vi "main(Test DQMH modules).vi"() -> ()   [LabVIEW 2018, in "Application.lvlib"] (continued)
              n418 = call "App enquece.vi"("command"=w959, "queue in"=w958) -> ("error out"=w960:errorcluster)  [unwired: 8 in, 1 out]
            }
            n419 = Merge Errors(w951, w949) -> (w950:errorcluster)
          }
          event "Test Channel 1": Value Change {
            n420 = event-data() -> ()  [unwired: 1 in, 1 out]
            n421 = Array Subset(array=w968, index=0, length=6) -> (w965:refnum<vi>[])
            n422 = for {
              tunnel: w965 -> [w977] mode=indexing
              n423 = property class="ColBox"(reference=w977, "Value"=u32 10000536 ("DRV 1")) -> ()  [unwired: 1 in, 2 out]
            }
            n424 = Build Array("Test Channel 1", "MEAS.AllRelaysOFF") -> (w972:string[])
            n425 = for {
              tunnel: [w981] -> w973 mode=indexing
              tunnel: w972 -> [w980] mode=indexing
              tunnel: w971 -> [w979]
              n426 = call "App enquece.vi"("command"=w980, "queue in"=w979) -> ("error out"=w981:errorcluster)  [unwired: 8 in, 1 out]
            }
            n427 = Merge Errors(w975, w973) -> (w974:errorcluster)
          }
          event "Test Channel 2": Value Change {
            n428 = event-data() -> ()  [unwired: 1 in, 1 out]
            n429 = Array Subset(array=w987, index=6, length=6) -> (w986:refnum<vi>[])
            n430 = for {
              tunnel: w986 -> [w998] mode=indexing
              n431 = property class="ColBox"(reference=w998, "Value"=u32 10000536 ("DRV 1")) -> ()  [unwired: 1 in, 2 out]
            }
            n432 = Build Array("Test Channel 2", "MEAS.AllRelaysOFF") -> (w993:string[])
            n433 = for {
              tunnel: [w1002] -> w994 mode=indexing
              tunnel: w993 -> [w1001] mode=indexing
              tunnel: w992 -> [w1000]
              n434 = call "App enquece.vi"("command"=w1001, "queue in"=w1000) -> ("error out"=w1002:errorcluster)  [unwired: 8 in, 1 out]
            }
            n435 = Merge Errors(w996, w994) -> (w995:errorcluster)
          }
          event "Test Channel 3": Value Change {
            n436 = event-data() -> ()  [unwired: 1 in, 1 out]
            n437 = Array Subset(array=w1007, index=12, length=6) -> (w1008:refnum<vi>[])
            n438 = for {
              tunnel: w1008 -> [w1019] mode=indexing
              n439 = property class="ColBox"(reference=w1019, "Value"=u32 10000536 ("DRV 1")) -> ()  [unwired: 1 in, 2 out]
            }
            n440 = Build Array("Test Channel 3", "MEAS.AllRelaysOFF") -> (w1014:string[])
            n441 = for {
              tunnel: [w1023] -> w1015 mode=indexing
              tunnel: w1014 -> [w1022] mode=indexing
              tunnel: w1013 -> [w1021]
              n442 = call "App enquece.vi"("command"=w1022, "queue in"=w1021) -> ("error out"=w1023:errorcluster)  [unwired: 8 in, 1 out]
            }
            n443 = Merge Errors(w1017, w1015) -> (w1016:errorcluster)
          }
          event "Test Channel 4": Value Change {
            n444 = event-data() -> ()  [unwired: 1 in, 1 out]
            n445 = Array Subset(array=w1028, index=18, length=6) -> (w1029:refnum<vi>[])
            n446 = for {
              tunnel: w1029 -> [w1040] mode=indexing
              n447 = property class="ColBox"(reference=w1040, "Value"=u32 10000536 ("DRV 1")) -> ()  [unwired: 1 in, 2 out]
            }
            n448 = Build Array("Test Channel 4", "MEAS.AllRelaysOFF") -> (w1035:string[])
            n449 = for {
              tunnel: [w1044] -> w1036 mode=indexing
              tunnel: w1035 -> [w1043] mode=indexing
              tunnel: w1034 -> [w1042]
              n450 = call "App enquece.vi"("command"=w1043, "queue in"=w1042) -> ("error out"=w1044:errorcluster)  [unwired: 8 in, 1 out]
            }
            n451 = Merge Errors(w1038, w1036) -> (w1037:errorcluster)
          }
          event "Test Channel 5": Value Change {
            n452 = event-data() -> ()  [unwired: 1 in, 1 out]
            n453 = Array Subset(array=w1049, index=24, length=6) -> (w1050:refnum<vi>[])
            n454 = for {
              tunnel: w1050 -> [w1061] mode=indexing
              n455 = property class="ColBox"(reference=w1061, "Value"=u32 10000536 ("DRV 1")) -> ()  [unwired: 1 in, 2 out]
            }
            n456 = Build Array("Test Channel 5", "MEAS.AllRelaysOFF") -> (w1056:string[])
            n457 = for {
              tunnel: [w1065] -> w1057 mode=indexing
              tunnel: w1056 -> [w1064] mode=indexing
              tunnel: w1055 -> [w1063]
              n458 = call "App enquece.vi"("command"=w1064, "queue in"=w1063) -> ("error out"=w1065:errorcluster)  [unwired: 8 in, 1 out]
            }
            n459 = Merge Errors(w1059, w1057) -> (w1058:errorcluster)
          }
          event "Test Channel 6": Value Change {
            n460 = event-data() -> ()  [unwired: 1 in, 1 out]
            n461 = Array Subset(array=w1070, index=30, length=6) -> (w1071:refnum<vi>[])
            n462 = for {
              tunnel: w1071 -> [w1082] mode=indexing
              n463 = property class="ColBox"(reference=w1082, "Value"=u32 10000536 ("DRV 1")) -> ()  [unwired: 1 in, 2 out]
            }
            n464 = Build Array("Test Channel 6", "MEAS.AllRelaysOFF") -> (w1077:string[])
            n465 = for {
              tunnel: [w1086] -> w1078 mode=indexing
              tunnel: w1077 -> [w1085] mode=indexing
              tunnel: w1076 -> [w1084]
              n466 = call "App enquece.vi"("command"=w1085, "queue in"=w1084) -> ("error out"=w1086:errorcluster)  [unwired: 8 in, 1 out]
            }
            n467 = Merge Errors(w1080, w1078) -> (w1079:errorcluster)
          }
          event "Test Channel 7": Value Change {
            n468 = event-data() -> ()  [unwired: 1 in, 1 out]
            n469 = Array Subset(array=w1091, index=36, length=6) -> (w1092:refnum<vi>[])
            n470 = for {
              tunnel: w1092 -> [w1103] mode=indexing
              n471 = property class="ColBox"(reference=w1103, "Value"=u32 10000536 ("DRV 1")) -> ()  [unwired: 1 in, 2 out]
            }
            n472 = Build Array("Test Channel 7", "MEAS.AllRelaysOFF") -> (w1099:string[])
            n473 = for {
              tunnel: [w1107] -> w1095 mode=indexing
              tunnel: w1099 -> [w1106] mode=indexing
              tunnel: w1098 -> [w1105]
              n474 = call "App enquece.vi"("command"=w1106, "queue in"=w1105) -> ("error out"=w1107:errorcluster)  [unwired: 8 in, 1 out]
            }
            n475 = Merge Errors(w1101, w1095) -> (w1100:errorcluster)
          }
          event "Test Channel 8": Value Change {
            n476 = event-data() -> ()  [unwired: 1 in, 1 out]
            n477 = Array Subset(array=w1112, index=42, length=6) -> (w1113:refnum<vi>[])
            n478 = for {
              tunnel: w1113 -> [w1124] mode=indexing
              n479 = property class="ColBox"(reference=w1124, "Value"=u32 10000536 ("DRV 1")) -> ()  [unwired: 1 in, 2 out]
            }
            n480 = Build Array("Test Channel 8", "MEAS.AllRelaysOFF") -> (w1119:string[])
            n481 = for {
              tunnel: [w1128] -> w1120 mode=indexing
              tunnel: w1119 -> [w1127] mode=indexing
              tunnel: w1118 -> [w1126]
              n482 = call "App enquece.vi"("command"=w1127, "queue in"=w1126) -> ("error out"=w1128:errorcluster)  [unwired: 8 in, 1 out]
            }
            n483 = Merge Errors(w1122, w1120) -> (w1121:errorcluster)
          }
          event "Test Channel 9": Value Change {
            n484 = event-data() -> ()  [unwired: 1 in, 1 out]
            n485 = Array Subset(array=w1133, index=48, length=6) -> (w1134:refnum<vi>[])
            n486 = for {
              tunnel: w1134 -> [w1145] mode=indexing
              n487 = property class="ColBox"(reference=w1145, "Value"=u32 10000536 ("DRV 1")) -> ()  [unwired: 1 in, 2 out]
            }
            n488 = Build Array("Test Channel 9", "MEAS.AllRelaysOFF") -> (w1140:string[])
            n489 = for {
              tunnel: [w1149] -> w1141 mode=indexing
              tunnel: w1140 -> [w1148] mode=indexing
              tunnel: w1139 -> [w1147]
              n490 = call "App enquece.vi"("command"=w1148, "queue in"=w1147) -> ("error out"=w1149:errorcluster)  [unwired: 8 in, 1 out]
            }
            n491 = Merge Errors(w1143, w1141) -> (w1142:errorcluster)
          }
          event "Test Channel 10": Value Change {
            n492 = event-data() -> ()  [unwired: 1 in, 1 out]
            n493 = Array Subset(array=w1154, index=54, length=6) -> (w1155:refnum<vi>[])
            n494 = for {
              tunnel: w1155 -> [w1166] mode=indexing
              n495 = property class="ColBox"(reference=w1166, "Value"=u32 10000536 ("DRV 1")) -> ()  [unwired: 1 in, 2 out]
            }
            n496 = Build Array("Test Channel 10", "MEAS.AllRelaysOFF") -> (w1161:string[])
            n497 = for {
              tunnel: [w1170] -> w1162 mode=indexing
              tunnel: w1161 -> [w1169] mode=indexing
              tunnel: w1160 -> [w1168]
              n498 = call "App enquece.vi"("command"=w1169, "queue in"=w1168) -> ("error out"=w1170:errorcluster)  [unwired: 8 in, 1 out]
            }
            n499 = Merge Errors(w1164, w1162) -> (w1163:errorcluster)
          }
          event User Event {
            n500 = event-data() -> ("Init?"=w1175:bool)  [unwired: 1 in]
            "DC Measure Module" <- w1175
            "Inst. 1" <- w1175
            n501 = disable-structure shown="LOGGING==TRUE" {
              disable-tunnel: w1178 -> [w1183 _]
              frame condition #0 (active) {
                n502 = Empty String/Path?(string/path=w1183) -> (empty?=w1189:bool)
                n503 = Select(t="Quece timeout", s=w1189, f=w1183) -> (s? t:f=w1187:string)
                n504 = Format Into String(format string=":%s", initial string=w1187, "DMM  Did  it") -> (resulting string=w1184:string)  [unwired: 1 in, 1 out]
                n505 = call "string log (SubVI).vi"("state Name"=w1184) -> ()  [unwired: 9 in, 2 out]
              }
              frame condition #1 {
              }
            }
            n506 = call "FGV Init phase.vi"("Boolean"=w1175) -> ("Init Completed?"=w1174:bool)  [unwired: 9 in, 1 out]
            n507 = case shown="True" w1174 {
              tunnel: w1173 -> [_ w1182]
              frame False {
              }
              frame True {
                n508 = call "App enquece.vi"("command"="INIT.Read DRV code", "queue in"=w1182) -> ()  [unwired: 8 in, 2 out]
              }
            }
          }
          event User Event {
            n509 = event-data() -> ("Init?"=w1193:bool)  [unwired: 1 in]
            "AC switches Module" <- w1193
            "Inst. 2" <- w1193
            n510 = disable-structure shown="LOGGING==TRUE" {
              disable-tunnel: w1198 -> [w1207 _]
              frame condition #0 (active) {
                n511 = Empty String/Path?(string/path=w1207) -> (empty?=w1213:bool)
                n512 = Select(t="Quece timeout", s=w1213, f=w1207) -> (s? t:f=w1211:string)
                n513 = Format Into String(format string=":%s", initial string=w1211, "MB01  Did  it") -> (resulting string=w1208:string)  [unwired: 1 in, 1 out]
                n514 = call "string log (SubVI).vi"("state Name"=w1208) -> ()  [unwired: 9 in, 2 out]
              }
              frame condition #1 {
              }
            }
            n515 = call "FGV Init phase.vi"("Boolean"=w1193) -> ("Init Completed?"=w1192:bool)  [unwired: 9 in, 1 out]
            n516 = case shown="True" w1192 {
              tunnel: w1191 -> [_ w1201]
              frame False {
              }
              frame True {
                n517 = call "App enquece.vi"("command"="INIT.Read DRV code", "queue in"=w1201) -> ()  [unwired: 8 in, 2 out]
              }
            }
            n518 = disable-structure shown="DEBUGGING==TRUE" {
              disable-tunnel: [w1203 w1206] -> w1197
              disable-tunnel: w1196 -> [w1203 w1205]
              frame condition #0 (active) {
              }
              frame condition #1 {
                n519 = call "Show Panel.vi"() -> ("error out"=w1204:errorcluster)  [unwired: 11 in]
                n520 = Merge Errors(w1205, w1204) -> (w1206:errorcluster)
              }
            }
          }
          event User Event {
            n521 = event-data() -> ("Init?"=w1218:bool)  [unwired: 1 in]
            "DC Switches Module" <- w1218
            "Inst. 3" <- w1218
            n522 = disable-structure shown="LOGGING==TRUE" {
              disable-tunnel: w1221 -> [w1226 _]
              frame condition #0 (active) {
                n523 = Empty String/Path?(string/path=w1226) -> (empty?=w1232:bool)
                n524 = Select(t="Quece timeout", s=w1232, f=w1226) -> (s? t:f=w1230:string)
                n525 = Format Into String(format string=":%s", initial string=w1230, "M054  Did  it") -> (resulting string=w1227:string)  [unwired: 1 in, 1 out]
                n526 = call "string log (SubVI).vi"("state Name"=w1227) -> ()  [unwired: 9 in, 2 out]
              }
              frame condition #1 {
              }
            }
            n527 = call "FGV Init phase.vi"("Boolean"=w1218) -> ("Init Completed?"=w1217:bool)  [unwired: 9 in, 1 out]
            n528 = case shown="True" w1217 {
              tunnel: w1216 -> [_ w1224]
              frame False {
              }
              frame True {
                n529 = call "App enquece.vi"("command"="INIT.Read DRV code", "queue in"=w1224) -> ()  [unwired: 8 in, 2 out]
              }
            }
          }
        }
      }
      frame "Apps.AutoMode" {
        # "Delay 1sec for Reset JIG execution Time"
        # "Check JIG trigger every 150ms"
        n530 = Wait (ms)(milliseconds to wait=u32 1000) -> ()  [unwired: 1 out]
      }
      frame "Apps.WaitingForTrigger" {
        n531 = call "App enquece.vi"("command"="MEAS.Read TRIGGER", "queue in"=w1247) -> ("error out"=w1245:errorcluster)  [unwired: 8 in, 1 out]
        n532 = Merge Errors(w1243, w1245) -> (w1244:errorcluster)
      }
      frame "Apps.UpdateStatus" {
        n533 = disable-structure shown="LOGGING==TRUE" {
          disable-tunnel: w1255 -> [w1268 _]
          frame condition #0 (active) {
            n534 = Empty String/Path?(string/path=w1268) -> (empty?=w1270:bool)
            n535 = Select(t="Quece timeout", s=w1270, f=w1268) -> (s? t:f=w1267:string)
            n536 = call "string log (SubVI).vi"("state Name"=w1267) -> ()  [unwired: 9 in, 2 out]
          }
          frame condition #1 {
          }
        }
        n537 = call "App enquece.vi"("command"="Apps.WaitForEvent", "queue in"=w1263) -> ("error out"=w1260:errorcluster)  [unwired: 8 in, 1 out]
        n538 = Merge Errors(w1256, w1260) -> (w1257:errorcluster)
      }
      frame "Apps.UI Update" {
        # "Update UI  6LED (channel)"
        n539 = disable-structure shown="LOGGING==TRUE" {
          disable-tunnel: w1274 -> [w1394 _]
          frame condition #0 (active) {
            n540 = Empty String/Path?(string/path=w1394) -> (empty?=w1396:bool)
            n541 = Select(t="Quece timeout", s=w1396, f=w1394) -> (s? t:f=w1393:string)
            n542 = call "string log (SubVI).vi"("state Name"=w1393) -> ()  [unwired: 9 in, 2 out]
          }
          frame condition #1 {
          }
        }
        n543 = Variant To Data(type="", Variant=w1272) -> (data=w1271:string)  [unwired: 1 in, 1 out]
        n544 = case shown="\"E\"" w1271 {
          tunnel: [w1295 w1303 w1321 w1339 w1357 w1375] -> w1280
          tunnel: w1278 -> [w1293 w1304 w1322 w1340 w1358 w1376]
          tunnel: w1277 -> [w1290 w1305 w1323 w1341 w1359 w1377]
          frame "", Default {
            w1287 = 6 ("length")
            n545 = call "FGV Driver Data.vi"("DUT channel (1-11)"=w1290, "FGV enum(Read)"=FGV_DRV_data."Process" ("FGV DRV data enum")) -> ("60 DRV data"=w1288:T15[])  [unwired: 6 in, 3 out]
            n546 = Decrement(x=w1290) -> (x-1=w1291:i32)
            n547 = Multiply(x=w1291, y=w1287) -> (x*y=w1289:i32)
            n548 = Array Subset(array=w1288, index=w1289, length=w1287) -> (w1286:T15[])
            n549 = Array Subset(array=w1293, index=w1289, length=w1287) -> (w1292:refnum<vi>[])
            n550 = for {
              tunnel: w1292 -> [w1298] mode=indexing
              tunnel: w1286 -> [w1297] mode=indexing
              tunnel: [w1296] -> w1295 mode=indexing
              n551 = Unbundle By Name(w1297) -> ("DRV Fail/Pass (T)"=w1301:bool)
              n552 = Select(t=u32 16711686 ("DRV 1"), s=w1301, f=u32 65309 ("DRV 1")) -> (s? t:f=w1302:u32)
              n553 = property class="ColBox"(reference=w1298, "Value"=w1302) -> (error out=w1296:errorcluster)  [unwired: 1 in, 1 out]
            }
          }
          frame "A" {
            w1306 = 1
            n554 = call "FGV Driver Data.vi"("DUT channel (1-11)"=w1305, "FGV enum(Read)"=FGV_DRV_data."Process" ("FGV DRV data enum")) -> ("60 DRV data"=w1309:T15[])  [unwired: 6 in, 3 out]
            n555 = Decrement(x=w1305) -> (x-1=w1311:i32)
            n556 = Multiply(x=w1311, y=6 ("length")) -> (x*y=w1310:i32)
            n557 = Array Subset(array=w1309, index=w1310, length=w1306) -> (w1307:T15[])
            n558 = Array Subset(array=w1304, index=w1310, length=w1306) -> (w1312:refnum<vi>[])
            n559 = for {
              tunnel: w1312 -> [w1316] mode=indexing
              tunnel: w1307 -> [w1315] mode=indexing
              tunnel: [w1314] -> w1303 mode=indexing
              n560 = Unbundle By Name(w1315) -> ("DRV Fail/Pass (T)"=w1319:bool)
              n561 = Select(t=u32 16711686 ("DRV 1"), s=w1319, f=u32 65309 ("DRV 1")) -> (s? t:f=w1320:u32)
              n562 = property class="ColBox"(reference=w1316, "Value"=w1320) -> (error out=w1314:errorcluster)  [unwired: 1 in, 1 out]
            }
          }
          frame "B" {
            w1324 = 2
            n563 = call "FGV Driver Data.vi"("DUT channel (1-11)"=w1323, "FGV enum(Read)"=FGV_DRV_data."Process" ("FGV DRV data enum")) -> ("60 DRV data"=w1327:T15[])  [unwired: 6 in, 3 out]
            n564 = Decrement(x=w1323) -> (x-1=w1329:i32)
            n565 = Multiply(x=w1329, y=6 ("length")) -> (x*y=w1328:i32)
            n566 = Array Subset(array=w1327, index=w1328, length=w1324) -> (w1325:T15[])
            n567 = Array Subset(array=w1322, index=w1328, length=w1324) -> (w1330:refnum<vi>[])
            n568 = for {
              tunnel: w1330 -> [w1334] mode=indexing
              tunnel: w1325 -> [w1333] mode=indexing
              tunnel: [w1332] -> w1321 mode=indexing
              n569 = Unbundle By Name(w1333) -> ("DRV Fail/Pass (T)"=w1337:bool)
              n570 = Select(t=u32 16711686 ("DRV 1"), s=w1337, f=u32 65309 ("DRV 1")) -> (s? t:f=w1338:u32)
              n571 = property class="ColBox"(reference=w1334, "Value"=w1338) -> (error out=w1332:errorcluster)  [unwired: 1 in, 1 out]
            }
          }
          frame "C" {
            w1342 = 3
            n572 = call "FGV Driver Data.vi"("DUT channel (1-11)"=w1341, "FGV enum(Read)"=FGV_DRV_data."Process" ("FGV DRV data enum")) -> ("60 DRV data"=w1345:T15[])  [unwired: 6 in, 3 out]
            n573 = Decrement(x=w1341) -> (x-1=w1347:i32)
            n574 = Multiply(x=w1347, y=6 ("length")) -> (x*y=w1346:i32)
            n575 = Array Subset(array=w1345, index=w1346, length=w1342) -> (w1343:T15[])
            n576 = Array Subset(array=w1340, index=w1346, length=w1342) -> (w1348:refnum<vi>[])
            n577 = for {
              tunnel: w1348 -> [w1352] mode=indexing
              tunnel: w1343 -> [w1351] mode=indexing
              tunnel: [w1350] -> w1339 mode=indexing
              n578 = Unbundle By Name(w1351) -> ("DRV Fail/Pass (T)"=w1355:bool)
              n579 = Select(t=u32 16711686 ("DRV 1"), s=w1355, f=u32 65309 ("DRV 1")) -> (s? t:f=w1356:u32)
              n580 = property class="ColBox"(reference=w1352, "Value"=w1356) -> (error out=w1350:errorcluster)  [unwired: 1 in, 1 out]
            }
          }
          frame "D" {
            w1360 = 4
            n581 = call "FGV Driver Data.vi"("DUT channel (1-11)"=w1359, "FGV enum(Read)"=FGV_DRV_data."Process" ("FGV DRV data enum")) -> ("60 DRV data"=w1363:T15[])  [unwired: 6 in, 3 out]
            n582 = Decrement(x=w1359) -> (x-1=w1365:i32)
            n583 = Multiply(x=w1365, y=6 ("length")) -> (x*y=w1364:i32)
            n584 = Array Subset(array=w1363, index=w1364, length=w1360) -> (w1361:T15[])
            n585 = Array Subset(array=w1358, index=w1364, length=w1360) -> (w1366:refnum<vi>[])
            n586 = for {
              tunnel: w1366 -> [w1370] mode=indexing
              tunnel: w1361 -> [w1369] mode=indexing
              tunnel: [w1368] -> w1357 mode=indexing
              n587 = Unbundle By Name(w1369) -> ("DRV Fail/Pass (T)"=w1373:bool)
              n588 = Select(t=u32 16711686 ("DRV 1"), s=w1373, f=u32 65309 ("DRV 1")) -> (s? t:f=w1374:u32)
              n589 = property class="ColBox"(reference=w1370, "Value"=w1374) -> (error out=w1368:errorcluster)  [unwired: 1 in, 1 out]
            }
          }
          frame "E" {
            w1378 = 5
            n590 = call "FGV Driver Data.vi"("DUT channel (1-11)"=w1377, "FGV enum(Read)"=FGV_DRV_data."Process" ("FGV DRV data enum")) -> ("60 DRV data"=w1381:T15[])  [unwired: 6 in, 3 out]
            n591 = Decrement(x=w1377) -> (x-1=w1383:i32)
            n592 = Multiply(x=w1383, y=6 ("length")) -> (x*y=w1382:i32)
            n593 = Array Subset(array=w1381, index=w1382, length=w1378) -> (w1379:T15[])
            n594 = Array Subset(array=w1376, index=w1382, length=w1378) -> (w1384:refnum<vi>[])
            n595 = for {
              tunnel: w1384 -> [w1388] mode=indexing
              tunnel: w1379 -> [w1387] mode=indexing
              tunnel: [w1386] -> w1375 mode=indexing
              n596 = Unbundle By Name(w1387) -> ("DRV Fail/Pass (T)"=w1391:bool)
              n597 = Select(t=u32 16711686 ("DRV 1"), s=w1391, f=u32 65309 ("DRV 1")) -> (s? t:f=w1392:u32)
              n598 = property class="ColBox"(reference=w1388, "Value"=w1392) -> (error out=w1386:errorcluster)  [unwired: 1 in, 1 out]
            }
          }
        }
        n599 = Merge Errors(w1281, w1280) -> (w1282:errorcluster)
      }
      frame "Apps.UI Update 1" {
        # "For Update UI 1 LED"
        n600 = disable-structure shown="LOGGING==TRUE" {
          disable-tunnel: w1411 -> [w1419 _]
          frame condition #0 (active) {
            n601 = Empty String/Path?(string/path=w1419) -> (empty?=w1421:bool)
            n602 = Select(t="Quece timeout", s=w1421, f=w1419) -> (s? t:f=w1418:string)
            n603 = call "string log (SubVI).vi"("state Name"=w1418) -> ()  [unwired: 9 in, 2 out]
          }
          frame condition #1 {
          }
        }
        n604 = call "FGV Driver Data.vi"("DUT channel (1-11)"=w1409, "FGV enum(Read)"=FGV_DRV_data."Process" ("FGV DRV data enum")) -> ("60 DRV data"=w1402:T15[])  [unwired: 6 in, 3 out]
        n605 = Decrement(x=w1397) -> (x-1=w1398:i32)
        n606 = Index Array(array=w1403, index=w1398) -> (element=w1400:refnum<vi>)
        n607 = Index Array(array=w1402, index=w1398) -> (element=w1401:T15)
        n608 = Unbundle By Name(w1401) -> ("DRV Fail/Pass (T)"=w1399:bool)
        n609 = Select(t=u32 16711686 ("DRV 1"), s=w1399, f=u32 65309 ("DRV 1")) -> (s? t:f=w1406:u32)
        n610 = property class="ColBox"(reference=w1400, "Value"=w1406) -> (error out=w1412:errorcluster)  [unwired: 1 in, 1 out]
        n611 = Merge Errors(w1413, w1412) -> (w1414:errorcluster)
      }
      frame "Apps.UI Update 2" {
        w1422 = "Test Completed!!!!"
        # "For Update PCB OK/NG (1 LED)"
        n612 = local read "Auto/Man"() -> (w1429:bool)
        n613 = disable-structure shown="LOGGING==TRUE" {
          disable-tunnel: w1441 -> [w1466 _]
          frame condition #0 (active) {
            n614 = Empty String/Path?(string/path=w1466) -> (empty?=w1468:bool)
            n615 = Select(t="Quece timeout", s=w1468, f=w1466) -> (s? t:f=w1465:string)
            n616 = call "string log (SubVI).vi"("state Name"=w1465) -> ()  [unwired: 9 in, 2 out]
          }
          frame condition #1 {
          }
        }
        n617 = case shown="True" w1429 {
          tunnel: w1434 -> [_ w1457]
          tunnel: [_ w1456] -> w1433
          frame False {
          }
          frame True {
            n618 = call "App enquece.vi"("command"="Apps.AutoMode", "queue in"=w1457) -> ("error out"=w1456:errorcluster)  [unwired: 8 in, 1 out]
          }
        }
        n619 = call "FGV DUT steps.vi"() -> ("Steps OUT"=w1427:string[])  [unwired: 11 in]
        n620 = Index Array(array=w1427, index=1) -> (element=w1428:string)
        n621 = Decimal String To Number(string=w1428) -> (number=w1425:i32)  [unwired: 2 in, 1 out]
        n622 = call "FGV Driver Data.vi"("error in (no error)"=w1433, "FGV enum(Read)"=FGV_DRV_data."Process" ("FGV DRV data enum")) -> ("error out"=w1440:errorcluster, "60 DRV data"=w1438:T15[])  [unwired: 6 in, 2 out]
        n623 = call "find Index and length.vi"("number of DRV"=w1425) -> ("length"=w1423:i32, "index"=w1424:i32)  [unwired: 8 in, 1 out]
        n624 = Array Subset(array=w1438, index=w1424, length=w1423) -> (w1431:T15[])
        n625 = for {
          tunnel: w1431 -> [w1470] mode=indexing
          tunnel: [w1469] -> w1447 mode=indexing
          n626 = Unbundle By Name(w1470) -> ("DRV Fail/Pass (T)"=w1469:bool)
        }
        n627 = control-ref of="DRV 61"() -> (w1446:refnum<vi>)
        n628 = Or Array Elements(Boolean array=w1447) -> (logical OR=w1445:bool)
        n629 = Select(t=u32 16711680 ("DRV 1"), s=w1445, f=u32 6618880 ("DRV 1")) -> (s? t:f=w1442:u32)
        n630 = property class="ColBox"(reference=w1446, error in=w1440, "Value"=w1442) -> (error out=w1439:errorcluster)  [unwired: 1 out]
        n631 = Merge Errors(w1454, w1439) -> (w1435:errorcluster)
        n632 = case shown="True" "Log report" {
          tunnel: w1431 -> [_ w1459]
          tunnel: w1430 -> [_ w1460]
          frame False {
          }
          frame True {
            # "Log trigger"
            n633 = To Variant(anything=w1459) -> (Variant=w1458:variant)
            n634 = Enqueue Element(queue=w1460, element=w1458) -> ()  [unwired: 2 in, 3 out]
          }
        }
        n635 = disable-structure shown="NO_HARDWARE==TRUE" {
          disable-tunnel: [w1461 w1464] -> w1436
          disable-tunnel: w1435 -> [w1461 w1464]
          frame condition #0 {
            n636 = Wait (ms)(milliseconds to wait=u32 2000) -> ()  [unwired: 1 out]
          }
          frame condition #1 (active) {
            n637 = Wait (ms)(milliseconds to wait=u32 20) -> ()  [unwired: 1 out]
          }
        }
        n638 = local write "Progress Status"(w1422) -> ()
      }
      frame "Apps.UI Update SC" {
        w1481 = "All Shorted Circuits"
        n639 = disable-structure shown="LOGGING==TRUE" {
          disable-tunnel: w1487 -> [w1502 _]
          frame condition #0 (active) {
            n640 = Empty String/Path?(string/path=w1502) -> (empty?=w1504:bool)
            n641 = Select(t="Quece timeout", s=w1504, f=w1502) -> (s? t:f=w1501:string)
            n642 = call "string log (SubVI).vi"("state Name"=w1501) -> ()  [unwired: 9 in, 2 out]
          }
          frame condition #1 {
          }
        }
        n643 = call "FGV DUT steps.vi"() -> ("Steps OUT"=w1474:string[])  [unwired: 11 in]
        n644 = Index Array(array=w1474, index=1) -> (element=w1476:string)
        n645 = Decimal String To Number(string=w1476) -> (number=w1475:i32)  [unwired: 2 in, 1 out]
        n646 = call "find Index and length.vi"("number of DRV"=w1475) -> ("length"=w1471:i32, "index"=w1472:i32)  [unwired: 8 in, 1 out]
        n647 = call "FGV Driver Data.vi"("FGV enum(Read)"=FGV_DRV_data."Read" ("FGV DRV data enum")) -> ("60 DRV data"=w1478:T15[])  [unwired: 7 in, 3 out]
        n648 = Array Subset(array=w1478, index=w1472, length=w1471) -> (w1477:T15[])
        n649 = Array Subset(array=w1480, index=w1472, length=w1471) -> (w1479:refnum<vi>[])
        n650 = for {
          tunnel: w1477 -> [w1511] mode=indexing
          tunnel: w1479 -> [w1506] mode=indexing
          tunnel: [w1505] -> w1485 mode=indexing
          n651 = Unbundle By Name(w1511) -> ("Shorted Circuit"=w1507:bool)
          n652 = Select(t=u32 16711680 ("DRV 1"), s=w1507, f=u32 6618880 ("DRV 1")) -> (s? t:f=w1510:u32)
          n653 = property class="ColBox"(reference=w1506, "Value"=w1510) -> (error out=w1505:errorcluster)  [unwired: 1 in, 1 out]
        }
        n654 = Merge Errors(w1485) -> (w1484:errorcluster)
        n655 = flat-sequence {
          tunnel: w1484 -> [w1497]
          tunnel: [w1497] -> w1483
          tunnel: w1483 -> [w1499]
          tunnel: [w1500] -> w1482
          tunnel: w1480 -> [w1498]
          frame #0 {
            n656 = Wait (ms)(milliseconds to wait=u32 500) -> ()  [unwired: 1 out]
          }
          frame #1 {
            n657 = call "reset DRV UI (SubVI).vi"("error in (no error)"=w1499, "Ref  in"=w1498) -> ("error out"=w1500:errorcluster)  [unwired: 8 in, 1 out]
          }
        }
        n658 = Merge Errors(w1495, w1482) -> (w1486:errorcluster)
        n659 = local write "Progress Status"(w1481) -> ()
      }
      frame "Timer Start" {
        n660 = flat-sequence {
          tunnel: [""] -> w1512
          frame #0 {
            n661 = call "FGV milisec (subVI).vi"() -> ()  [unwired: 11 in, 1 out]
          }
        }
        n662 = local write "elapsed Time"(w1512) -> ()
      }
      frame "Timer Stop" {
        n663 = flat-sequence {
          tunnel: [w1537] -> w1527
          tunnel: w1528 -> [w1537]
          tunnel: [w1536] -> w1526
          frame #0 {
            n664 = call "FGV milisec (subVI).vi"() -> ("Elased Time (ms)"=w1536:u32)  [unwired: 11 in]
          }
        }
        n665 = Format Into String(initial string="t = ", w1526) -> (resulting string=w1524:string)  [unwired: 2 in, 1 out]
        n666 = Concatenate Strings(w1524, "  [ms] " ("initial string")) -> (→"elapsed Time":string)
      }
      frame "WaitFor" {
        n667 = flat-sequence {
          tunnel: [w1547] -> w1538
          tunnel: w1539 -> [w1547]
          frame #0 {
            n668 = Wait (ms)(milliseconds to wait="wait for (ms)") -> ()  [unwired: 1 out]
          }
        }
      }
      frame "WaitForA" {
        n669 = flat-sequence {
          tunnel: [w1563] -> w1549
          tunnel: w1550 -> [w1563]
          frame #0 {
            n670 = local read "wait for (ms)"() -> (w1561:u32)
            n671 = Multiply(x=u32 230, y=u32 1) -> (x*y=w1562:u32)
            n672 = Subtract(x=w1561, y=w1562) -> (x-y=w1560:u32)
            n673 = Wait (ms)(milliseconds to wait=w1560) -> ()  [unwired: 1 out]
          }
        }
      }
      frame "WaitForB" {
        n674 = flat-sequence {
          tunnel: [w1578] -> w1564
          tunnel: w1565 -> [w1578]
          frame #0 {
            n675 = local read "wait for (ms)"() -> (w1576:u32)
            n676 = Multiply(x=u32 230, y=u32 2) -> (x*y=w1577:u32)
            n677 = Subtract(x=w1576, y=w1577) -> (x-y=w1575:u32)
            n678 = Wait (ms)(milliseconds to wait=w1575) -> ()  [unwired: 1 out]
          }
        }
      }
      frame "WaitForC" {
        n679 = flat-sequence {
          tunnel: [w1593] -> w1579
          tunnel: w1580 -> [w1593]
          frame #0 {
            n680 = local read "wait for (ms)"() -> (w1591:u32)
            n681 = Multiply(x=u32 230, y=u32 3) -> (x*y=w1592:u32)
            n682 = Subtract(x=w1591, y=w1592) -> (x-y=w1590:u32)
            n683 = Wait (ms)(milliseconds to wait=w1590) -> ()  [unwired: 1 out]
          }
        }
      }
      frame "WaitForD" {
        n684 = flat-sequence {
          tunnel: [w1608] -> w1594
          tunnel: w1595 -> [w1608]
          frame #0 {
            n685 = local read "wait for (ms)"() -> (w1606:u32)
            n686 = Multiply(x=u32 230, y=u32 4) -> (x*y=w1607:u32)
            n687 = Subtract(x=w1606, y=w1607) -> (x-y=w1605:u32)
            n688 = Wait (ms)(milliseconds to wait=w1605) -> ()  [unwired: 1 out]
          }
        }
      }
      frame "WaitForE" {
        n689 = flat-sequence {
          tunnel: [w1623] -> w1609
          tunnel: w1610 -> [w1623]
          frame #0 {
            n690 = local read "wait for (ms)"() -> (w1621:u32)
            n691 = Multiply(x=u32 230, y=u32 5) -> (x*y=w1622:u32)
            n692 = Subtract(x=w1621, y=w1622) -> (x-y=w1620:u32)
            n693 = Wait (ms)(milliseconds to wait=w1620) -> ()  [unwired: 1 out]
          }
        }
      }
      frame "Apps.Exit" {
        w1628 = TRUE
        n694 = disable-structure shown="LOGGING==TRUE" {
          disable-tunnel: w1625 -> [w1643 _]
          frame condition #0 (active) {
            n695 = Empty String/Path?(string/path=w1643) -> (empty?=w1645:bool)
            n696 = Select(t="Quece timeout", s=w1645, f=w1643) -> (s? t:f=w1642:string)
            n697 = call "string log (SubVI).vi"("state Name"=w1642) -> ()  [unwired: 9 in, 2 out]
          }
          frame condition #1 {
          }
        }
        n698 = call "Application Name--constant.vi"() -> ("Application Name"=w1629:string)  [unwired: 11 in]
        n699 = call "Stop Module.vi"("Wait for Module to Stop? (F)"=w1628, "Origin"=w1629) -> ("error out"=w1637:errorcluster)  [unwired: 9 in]
        n700 = call "Stop Module.vi"("Wait for Module to Stop? (F)"=w1628, "Origin"=w1629) -> ("error out"=w1636:errorcluster)  [unwired: 9 in]
        n701 = call "Stop Module.vi"("Wait for Module to Stop? (F)"=w1628, "Origin"=w1629) -> ("error out"=w1635:errorcluster)  [unwired: 9 in]
        n702 = call "Stop Module.vi"("Wait for Module to stop? (F)"=w1628, "Origin"=w1629, "Module ID"=-1) -> ("error out"=w1631:errorcluster)  [unwired: 8 in]
        n703 = Merge Errors(w1633, w1637, w1636, w1635, w1631) -> (w1634:errorcluster)
      }
      frame "Apps.Error Handler" {
        w1654 = TRUE  # Priority Enquece
        n704 = disable-structure shown="LOGGING==TRUE" {
          disable-tunnel: w1647 -> [w1663 _]
          frame condition #0 (active) {
            n705 = Empty String/Path?(string/path=w1663) -> (empty?=w1665:bool)
            n706 = Select(t="Quece timeout", s=w1665, f=w1663) -> (s? t:f=w1662:string)
            n707 = call "string log (SubVI).vi"("state Name"=w1662) -> ()  [unwired: 9 in, 2 out]
          }
          frame condition #1 {
          }
        }
        n708 = call <vilib>:"Simple Error Handler.vi"("error in (no error)"=w1661) -> ("error out"=w1656:errorcluster)  [unwired: 4 in, 4 out]
        n709 = flat-sequence {
          tunnel: w1656 -> [_]
          tunnel: [w1666] -> w1648
          frame #0 {
            n710 = xnode "Error Ring"() -> ("error out"=w1666:errorcluster)
          }
        }
        n711 = call "App enquece.vi"("Priority Enquece"=w1654, "command"="Apps.Exit", "queue in"=w1655) -> ("error out"=w1653:errorcluster)  [unwired: 7 in, 1 out]
        n712 = Merge Errors(w1648, w1653) -> (w1649:errorcluster)
      }
      frame "INIT.Init FGV" {
        n713 = call "FGV_HoldingRegs.vi"("FGV_enum"=FGV_enum."Init FGV") -> ("error out"=w1673:errorcluster)  [unwired: 8 in, 2 out]
        n714 = call "string log (SubVI).vi"("error in (no error)"=w1673, "Enum(log)"=enum16{"Init", "Log", "Read", "Clear"}."Init") -> ("error out"=w1674:errorcluster)  [unwired: 8 in, 1 out]
        n715 = call "FGV Driver Data.vi"("error in (no error)"=w1674, "FGV enum(Read)"=FGV_DRV_data."Init" ("FGV DRV data enum")) -> ("error out"=w1671:errorcluster)  [unwired: 6 in, 3 out]
        n716 = call "FGV Init phase.vi"("error in (no error)"=w1671, "FGV Enum"=enum16{"Init", "Check"}."Init") -> ("error out"=w1669:errorcluster)  [unwired: 8 in, 1 out]
        n717 = flat-sequence {
          tunnel: [w1686] -> w1670
          tunnel: w1669 -> [w1686]
          frame #0 {
            n718 = Initialize Array(FALSE, 6 ("dimension size"), 10 ("dimension size")) -> (w1690:bool[][])
            n719 = local write "Auto/Man"(FALSE) -> ()
            n720 = local write "EMIC connected"(bool[] [FALSE, FALSE, FALSE, FALSE, FALSE, FALSE] ("Array")) -> ()
            n721 = local write "Short DRV"(w1690) -> ()
          }
        }
        n722 = Merge Errors(w1685, w1670) -> (w1675:errorcluster)
      }
      frame "INIT.Read HW config" {
        n723 = disable-structure shown="LOGGING==TRUE" {
          disable-tunnel: w1705 -> [w1731 _]
          frame condition #0 (active) {
            n724 = Empty String/Path?(string/path=w1731) -> (empty?=w1733:bool)
            n725 = Select(t="Quece timeout", s=w1733, f=w1731) -> (s? t:f=w1730:string)
            n726 = call "string log (SubVI).vi"("state Name"=w1730) -> ()  [unwired: 9 in, 2 out]
          }
          frame condition #1 {
          }
        }
        n727 = call <vilib>:"Application Directory.vi"() -> ("Application Directory"=w1700:path)
        n728 = Build Path(base path=w1700, name or relative path="config") -> (appended path=w1699:path)
        n729 = call "HW Config.vi"("start path"=w1699) -> ("error out"=w1706:errorcluster, "HW config 2"=w1713:T7)  [unwired: 9 in]
        n730 = Bundle By Name(cluster=w1714, "HW config 2"=w1713) -> (w1712:cluster{"HW config 2":T7})
        n731 = invoke class="VI" method="FP.Open"(error in=w1706, "State"=T17."Minimized") -> (error out=w1695:errorcluster)  [unwired: 3 in, 4 out]
        n732 = call "Login.vi"("error in (no error)"=w1695) -> ("error out"=w1697:errorcluster, "Login Successed"=w1698:bool, "UserName"=w1694:string)  [unwired: 8 in]
        n733 = call "FGV _Operator Name.vi"("Enum"=enum16{"Write", "Read"}."Write", "Operator Name in"=w1694) -> ()  [unwired: 9 in, 1 out]
        n734 = case shown="True" w1698 {
          tunnel: w1702 -> [w1724 _]
          tunnel: w1697 -> [w1721 w1726]
          tunnel: [w1720 w1727] -> w1707
          frame False {
            n735 = call "string log (SubVI).vi"("Enum(log)"=enum16{"Init", "Log", "Read", "Clear"}."Init") -> ("error out"=w1719:errorcluster)  [unwired: 9 in, 1 out]
            n736 = call "App enquece.vi"("Priority Enquece"=TRUE, "error in (no error)"=w1721, "command"="Apps.Exit", "queue in"=w1724) -> ("error out"=w1720:errorcluster)  [unwired: 6 in, 1 out]
            n737 = call "inst.InitialiseFGV.vi"("error in (no error)"=w1719) -> ()  [unwired: 10 in, 1 out]
          }
          frame True {
            n738 = invoke class="VI" method="FP.Open"(error in=w1726, "State"=T17."Standard") -> (error out=w1727:errorcluster)  [unwired: 3 in, 4 out]
          }
        }
        n739 = Merge Errors(w1717, w1707) -> (w1708:errorcluster)
        n740 = disable-structure shown="RUN_TIME_ENGINE==True" {
          disable-tunnel: ["Under Development" ("version") "v5.0 Released"] -> w1704
          frame condition #0 (active) {
          }
          frame condition #1 {
          }
        }
        "version" <- w1704
      }
      frame "INIT.Read DRV code" {
        n741 = disable-structure shown="LOGGING==TRUE" {
          disable-tunnel: w1762 -> [w1795 _]
          frame condition #0 (active) {
            n742 = Empty String/Path?(string/path=w1795) -> (empty?=w1797:bool)
            n743 = Select(t="Quece timeout", s=w1797, f=w1795) -> (s? t:f=w1794:string)
            n744 = call "string log (SubVI).vi"("state Name"=w1794) -> ()  [unwired: 9 in, 2 out]
          }
          frame condition #1 {
          }
        }
        n745 = invoke class="VI" method="FP.Open"("State"=T17."Minimized") -> (error out=w1756:errorcluster)  [unwired: 4 in, 4 out]
        n746 = call "ReadDriverParameters.vi"("error in (no error)"=w1756) -> ("error out"=w1754:errorcluster, "DRV stand"=w1745:T16)  [unwired: 9 in]
        n747 = invoke class="VI" method="FP.Open"(error in=w1754, "State"=T17."Standard") -> (error out=w1758:errorcluster)  [unwired: 3 in, 4 out]
        n748 = Merge Errors(w1763, w1758) -> (w1764:errorcluster)
        n749 = call "FGV DRV stand.vi"("Enum(read)"=enum16{"Write", "Read"}."Write" ("Enum"), "DRV stand  in"=w1745) -> ("Sub-Test.DCV"=w1734:bool, "DRV stand out"=w1744:T16)  [unwired: 8 in]
        n750 = Unbundle By Name(w1744) -> ("SAP ID"=w1751:string, "Name"=w1752:string)
        "DUT Name" <- w1752
        n751 = call "FGV SapID & Name.vi"("Enum"=enum16{"Read", "Write"}."Write", "Name"=w1752, "SAP ID"=w1751) -> ("SAP ID out"=w1748:string)  [unwired: 7 in, 1 out]
        n752 = case shown="True" w1734 {
          tunnel: w1761 -> [_ w1787]
          tunnel: [_ w1774] -> w1753
          tunnel: w1744 -> [_ w1773]
          tunnel: ["HV-60D ready!!!!!!!!!!!!!!!!" w1772] -> w1747
          tunnel: w1746 -> [_ w1772]
          frame False {
          }
          frame True {
            w1786 = u8 2 items=["SLOW", "MID", "FAST"] ("Detector Rate")
            # "Convert from [mA] to [A]"
            n753 = Unbundle By Name(w1773) -> ("DC characteristics.Voltage.Max"=w1778:dbl, "DC characteristics.Current.Max"=w1793:dbl)
            n754 = Divide(x=w1793, y=1000.0) -> (x/y=w1775:dbl)
            n755 = Bundle By Name(cluster=T19 {"DMM config cluster"={"DCV range"=0.0, "DCI range"=0.0, "Detector Rate"=0}, "mux2-1(DMM I) encode"=enum."DMM I (0.5)"} ("DMM all config"), "DMM config cluster.DCV range"=w1778, "DMM config cluster.DCI range"=w1775, "DMM config cluster.Detector Rate"=w1786) -> (w1790:T19)
            n756 = Greater?(x=w1775, y=0.5) -> (0:w1776:bool)
            n757 = To Variant(anything=w1790) -> (Variant=w1789:variant)
            n758 = Select(t=enum16{"DMM I (0.5)", "DMM I (12)"}."DMM I (12)" ("mux2-1(DMM I) encode 2"), s=w1776, f=enum16{"DMM I (0.5)", "DMM I (12)"}."DMM I (0.5)" ("mux2-1(DMM I) encode 2")) -> (s? t:f=w1782:enum16{"DMM I (0.5)", "DMM I (12)"})
            n759 = call "App enquece.vi"("command data"=w1789, "command"="MEAS.Set DMM config", "queue in"=w1787) -> ("error out"=w1779:errorcluster, "Queue out"=w1783:refnum<queue>)  [unwired: 7 in]
            n760 = To Variant(anything=w1782) -> (Variant=w1784:variant)
            n761 = call "App enquece.vi"("error in (no error)"=w1779, "command data"=w1784, "command"="MEAS.Sel Input Current", "queue in"=w1783) -> ("error out"=w1774:errorcluster)  [unwired: 6 in, 1 out]
          }
        }
        n762 = call "FGV DUT steps.vi"("Enum(read)"=enum16{"write", "read"}."write" ("Enum"), "SapID"=w1748) -> ("Steps OUT"=w1740:string[])  [unwired: 9 in]
        n763 = Index Array(array=w1740, index #1=0 ("index")) -> (element #1=→"SAP ID":string, element #2=→"#DRV":string, element #3=w1735:string)  [unwired: 2 in]
        n764 = Decimal String To Number(string=w1735) -> (number=w1742:i32)  [unwired: 2 in, 1 out]
        n765 = To Unsigned Long Integer(number=w1742) -> (unsigned 32bit integer=w1741:u32)
        n766 = local write "wait for (ms)"(w1741) -> ()
        n767 = Array Subset(array=w1740, index=3) -> (→"List of Actions":string[])  [unwired: 1 in]
        n768 = Merge Errors(w1764, w1753) -> (w1760:errorcluster)
      }
      frame "INIT.Call DMM module" {
        n769 = disable-structure shown="LOGGING==TRUE" {
          disable-tunnel: w1799 -> [w1817 _]
          frame condition #0 (active) {
            n770 = Empty String/Path?(string/path=w1817) -> (empty?=w1819:bool)
            n771 = Select(t="Quece timeout", s=w1819, f=w1817) -> (s? t:f=w1816:string)
            n772 = call "string log (SubVI).vi"("state Name"=w1816) -> ()  [unwired: 9 in, 2 out]
          }
          frame condition #1 {
          }
        }
        n773 = Unbundle By Name(w1810) -> ("HW config 2.DMM"=w1809:string)
        n774 = Type Cast(type=refnum<visa-resource-name> refnum ("VISA resource name 2"), x=w1809) -> (*(type *) &x=w1807:refnum<visa-resource-name>)
        n775 = call "Start Module.vi"("VISA resource name 2"=w1807) -> ("error out"=w1812:errorcluster, "Wait for Event Sync?"=w1806:bool, "DMM Module Broadcast Events"=w1805:T13)  [unwired: 7 in, 1 out]
        n776 = register-events(reference=w1813, w1805) -> (reference out=w1814:refnum<event-registration>)  [unwired: 5 in, 1 out]
        n777 = call "Synchronize Module Events.vi"("error in"=w1812, "Wait for Event Sync?"=w1806) -> ("error out"=w1811:errorcluster)  [unwired: 9 in]
        n778 = Merge Errors(w1800, w1811) -> (w1801:errorcluster)
      }
      frame "INIT.Call MUX module" {
        n779 = disable-structure shown="LOGGING==TRUE" {
          disable-tunnel: w1821 -> [w1839 _]
          frame condition #0 (active) {
            n780 = Empty String/Path?(string/path=w1839) -> (empty?=w1841:bool)
            n781 = Select(t="Quece timeout", s=w1841, f=w1839) -> (s? t:f=w1838:string)
            n782 = call "string log (SubVI).vi"("state Name"=w1838) -> ()  [unwired: 9 in, 2 out]
          }
          frame condition #1 {
          }
        }
        n783 = Unbundle By Name(w1833) -> ("HW config 2.mux"=w1832:string)
        n784 = Type Cast(type=refnum<visa-resource-name> refnum ("VISA resource name"), x=w1832) -> (*(type *) &x=w1831:refnum<visa-resource-name>)
        n785 = call "Start Module.vi"("VISA resource name"=w1831) -> ("error out"=w1834:errorcluster, "Wait for Event Sync?"=w1828:bool, "Switches Module Broadcast Events"=w1829:T11)  [unwired: 7 in, 1 out]
        n786 = register-events(reference=w1835, w1829) -> (reference out=w1836:refnum<event-registration>)  [unwired: 5 in, 1 out]
        n787 = call "Synchronize Module Events.vi"("error in"=w1834, "Wait for Event Sync?"=w1828) -> ("error out"=w1827:errorcluster)  [unwired: 9 in]
        n788 = Merge Errors(w1822, w1827) -> (w1823:errorcluster)
      }
      frame "INIT.Call DEMUX module" {
        n789 = disable-structure shown="LOGGING==TRUE" {
          disable-tunnel: w1844 -> [w1861 _]
          frame condition #0 (active) {
            n790 = Empty String/Path?(string/path=w1861) -> (empty?=w1863:bool)
            n791 = Select(t="Quece timeout", s=w1863, f=w1861) -> (s? t:f=w1860:string)
            n792 = call "string log (SubVI).vi"("state Name"=w1860) -> ()  [unwired: 9 in, 2 out]
          }
          frame condition #1 {
          }
        }
        n793 = Unbundle By Name(w1855) -> ("HW config 2.demux"=w1854:string)
        n794 = Type Cast(type=refnum<visa-resource-name> refnum ("COMport name"), x=w1854) -> (*(type *) &x=w1853:refnum<visa-resource-name>)
        n795 = call "Start Module.vi"("COMport name"=w1853) -> ("error out"=w1856:errorcluster, "Wait for Event Sync?"=w1842:bool, "MB 01 switches Module Broadcast Events"=w1851:T12)  [unwired: 7 in, 1 out]
        n796 = register-events(reference=w1857, w1851) -> (reference out=w1858:refnum<event-registration>)  [unwired: 5 in, 1 out]
        n797 = call "Synchronize Module Events.vi"("error in"=w1856, "Wait for Event Sync?"=w1842) -> ("error out"=w1850:errorcluster)  [unwired: 9 in]
        n798 = Merge Errors(w1845, w1850) -> (w1846:errorcluster)
      }
      frame "INIT.Call EMIC modules" {
        n799 = disable-structure shown="LOGGING==TRUE" {
          disable-tunnel: w1867 -> [w1884 _]
          frame condition #0 (active) {
            n800 = Empty String/Path?(string/path=w1884) -> (empty?=w1886:bool)
            n801 = Select(t="Quece timeout", s=w1886, f=w1884) -> (s? t:f=w1883:string)
            n802 = call "string log (SubVI).vi"("state Name"=w1883) -> ()  [unwired: 9 in, 2 out]
          }
          frame condition #1 {
          }
        }
        n803 = Unbundle By Name(w1874) -> ("HW config 2.eMIC1"=w1881:string, "HW config 2.eMIC2"=w1880:string, "HW config 2.eMIC3"=w1879:string, "HW config 2.eMIC4"=w1878:string, "HW config 2.eMIC5"=w1877:string, "HW config 2.eMIC6"=w1876:string)
        n804 = Build Array(w1881, w1880, w1879, w1878, w1877, w1876) -> (w1865:string[])
        n805 = for {
          shift-right: [w1896] -> w1873
          shift-left: w1875 -> [w1894]
          tunnel: w1865 -> [w1895] mode=indexing
          tunnel: [w1888] -> w1871 mode=indexing
          n806 = Type Cast(type=refnum<visa-resource-name> refnum ("VISA resource name"), x=w1895) -> (*(type *) &x=w1892:refnum<visa-resource-name>)
          n807 = call "Start Module.vi"("VISA resource name"=w1892) -> ("error out"=w1889:errorcluster, "Wait for Event Sync?"=w1887:bool, "CE14_v2 Broadcast Events"=w1891:T10, "Module ID"=w1890:i32)  [unwired: 7 in]
          n808 = register-events(reference=w1894, w1891) -> (reference out=w1896:refnum<event-registration>)  [unwired: 5 in, 1 out]
          n809 = call "Synchronize Module Events.vi"("error in"=w1889, "Wait for Event Sync?"=w1887, "Module ID in"=w1890) -> ("error out"=w1888:errorcluster)  [unwired: 7 in, 1 out]
        }
        n810 = Merge Errors(w1868, w1871) -> (w1866:errorcluster)
      }
      frame "INIT.Open COM DMM" {
        n811 = disable-structure shown="LOGGING==TRUE" {
          disable-tunnel: w1900 -> [w1912 _]
          frame condition #0 (active) {
            n812 = Empty String/Path?(string/path=w1912) -> (empty?=w1914:bool)
            n813 = Select(t="Quece timeout", s=w1914, f=w1912) -> (s? t:f=w1911:string)
            n814 = call "string log (SubVI).vi"("state Name"=w1911) -> ()  [unwired: 9 in, 2 out]
          }
          frame condition #1 {
          }
        }
        n815 = call "DMM connect and reset.vi"() -> ("error out"=w1904:errorcluster)  [unwired: 11 in]
        n816 = Merge Errors(w1901, w1904) -> (w1898:errorcluster)
        n817 = flat-sequence {
          tunnel: [w1910] -> w1899
          tunnel: w1898 -> [w1910]
          frame #0 {
            n818 = Wait (ms)(milliseconds to wait=u32 70) -> ()  [unwired: 1 out]
          }
        }
      }
      frame "INIT.Open COM MUX" {
        n819 = disable-structure shown="LOGGING==TRUE" {
          disable-tunnel: w1918 -> [w1930 _]
          frame condition #0 (active) {
            n820 = Empty String/Path?(string/path=w1930) -> (empty?=w1932:bool)
            n821 = Select(t="Quece timeout", s=w1932, f=w1930) -> (s? t:f=w1929:string)
            n822 = call "string log (SubVI).vi"("state Name"=w1929) -> ()  [unwired: 9 in, 2 out]
          }
          frame condition #1 {
          }
        }
        n823 = call "inst.Open.vi"() -> ("error out"=w1924:errorcluster)  [unwired: 11 in]
        n824 = Merge Errors(w1919, w1924) -> (w1916:errorcluster)
        n825 = flat-sequence {
          tunnel: [w1928] -> w1917
          tunnel: w1916 -> [w1928]
          frame #0 {
            n826 = Wait (ms)(milliseconds to wait=u32 70) -> ()  [unwired: 1 out]
          }
        }
      }
      frame "INIT.Open COM DEMUX" {
        n827 = disable-structure shown="LOGGING==TRUE" {
          disable-tunnel: w1936 -> [w1948 _]
          frame condition #0 (active) {
            n828 = Empty String/Path?(string/path=w1948) -> (empty?=w1950:bool)
            n829 = Select(t="Quece timeout", s=w1950, f=w1948) -> (s? t:f=w1947:string)
            n830 = call "string log (SubVI).vi"("state Name"=w1947) -> ()  [unwired: 9 in, 2 out]
          }
          frame condition #1 {
          }
        }
        n831 = call "MB01 Open.vi"() -> ("error out"=w1941:errorcluster)  [unwired: 11 in]
        n832 = Merge Errors(w1937, w1941) -> (w1934:errorcluster)
        n833 = flat-sequence {
          tunnel: [w1946] -> w1935
          tunnel: w1934 -> [w1946]
          frame #0 {
            n834 = Wait (ms)(milliseconds to wait=u32 70) -> ()  [unwired: 1 out]
          }
        }
      }
      frame "INIT.Open COM EMIC" {
        n835 = disable-structure shown="LOGGING==TRUE" {
          disable-tunnel: w1954 -> [w1967 _]
          frame condition #0 (active) {
            n836 = Empty String/Path?(string/path=w1967) -> (empty?=w1969:bool)
            n837 = Select(t="Quece timeout", s=w1969, f=w1967) -> (s? t:f=w1966:string)
            n838 = call "string log (SubVI).vi"("state Name"=w1966) -> ()  [unwired: 9 in, 2 out]
          }
          frame condition #1 {
          }
        }
        n839 = call "Connect to CE14.vi"("Module ID"=-1) -> ("error out"=w1959:errorcluster)  [unwired: 10 in]
        n840 = Merge Errors(w1955, w1959) -> (w1952:errorcluster)
        n841 = flat-sequence {
          tunnel: [w1965] -> w1953
          tunnel: w1952 -> [w1965]
          frame #0 {
            n842 = Wait (ms)(milliseconds to wait=u32 70) -> ()  [unwired: 1 out]
          }
        }
      }
      frame "MEAS.Read EMIC connected" {
        n843 = disable-structure shown="LOGGING==TRUE" {
          disable-tunnel: w1987 -> [w2003 _]
          frame condition #0 (active) {
            n844 = Empty String/Path?(string/path=w2003) -> (empty?=w2005:bool)
            n845 = Select(t="Quece timeout", s=w2005, f=w2003) -> (s? t:f=w2002:string)
            n846 = call "string log (SubVI).vi"("state Name"=w2002) -> ()  [unwired: 9 in, 2 out]
          }
